vi "Yellow_Alarm_Counter.vi"(9 "Counter In":i32, 10 "Yellow Alarm":bool) -> (1 "Counter Out":i32, 2 "Counter Complete":bool)   [LabVIEW 2014]
panel:
  out "T Stoic Yellow \nMin Alarm":bool
  out "T Stoic Yellow \nMax Alarm":bool
  out "T Max Yellow\n Min Alarm":bool
  out "T Max Yellow \nMax Alarm":bool
  # "Yellow Alarm Counter Vi"
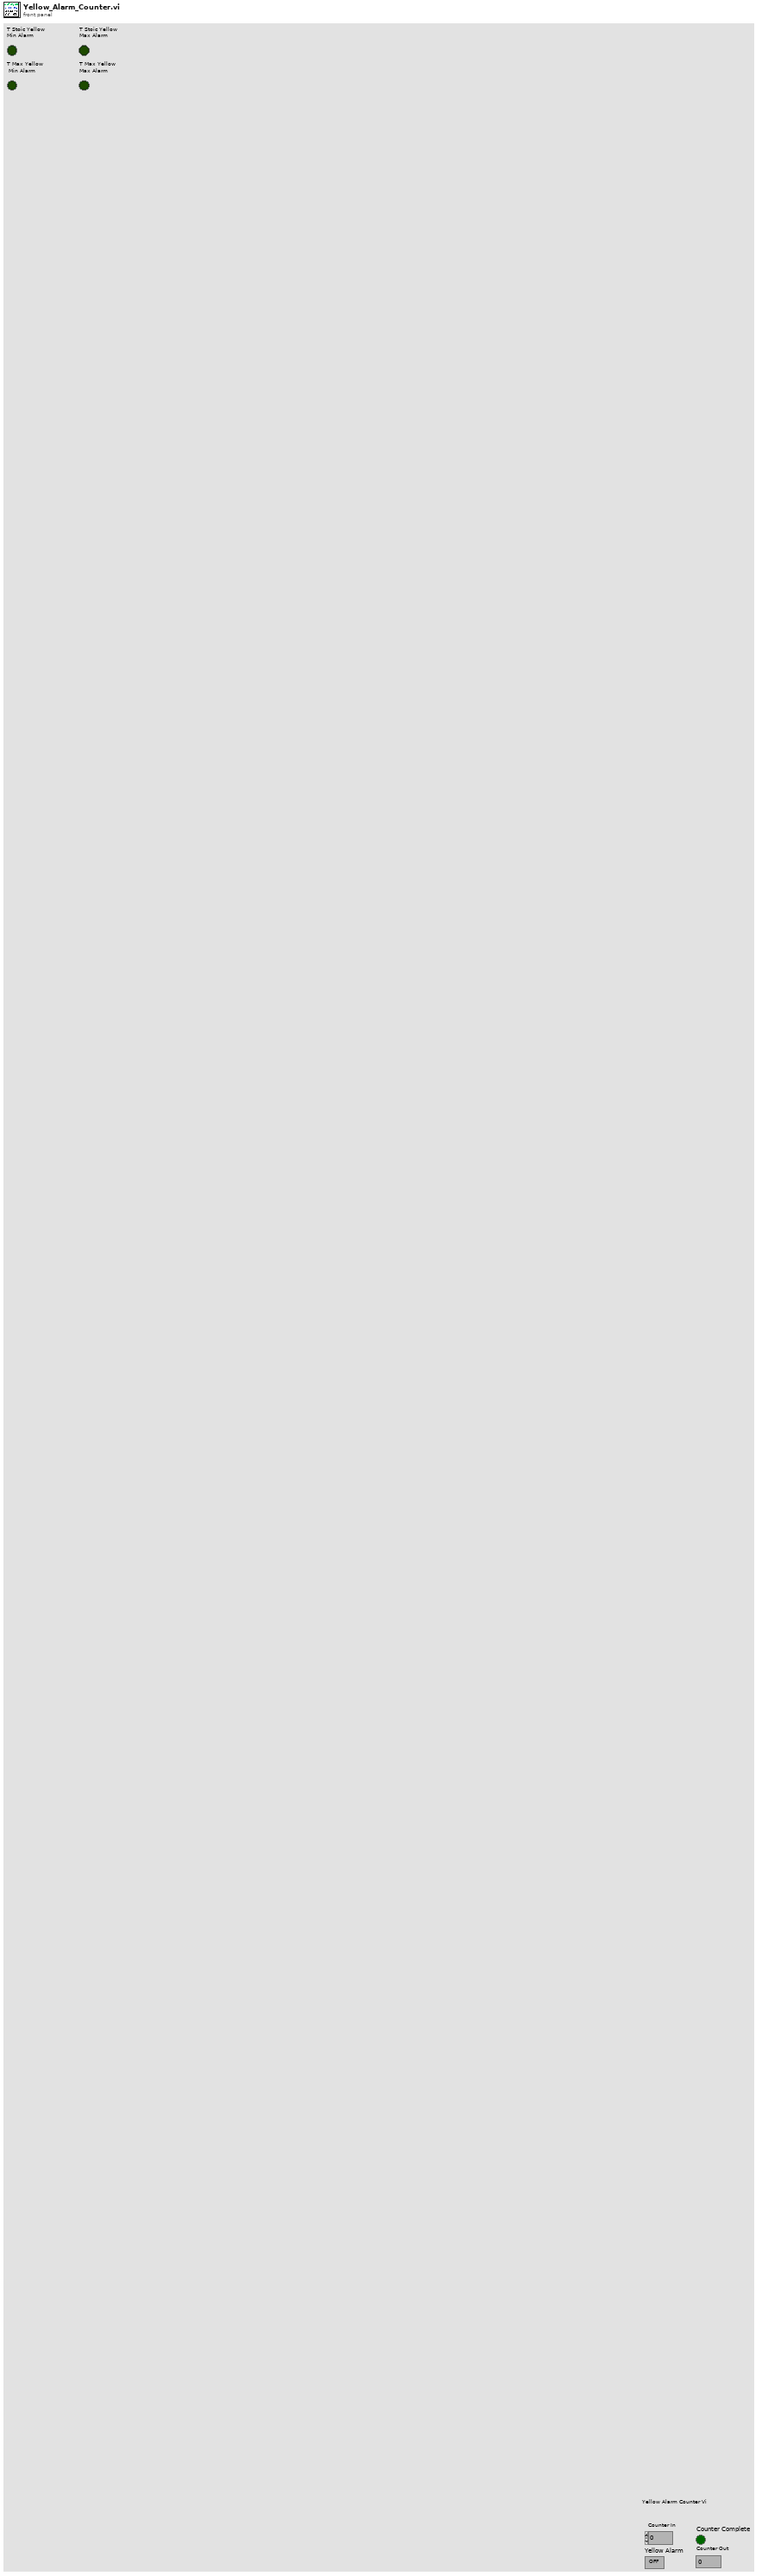
[diagram p1: front panel]
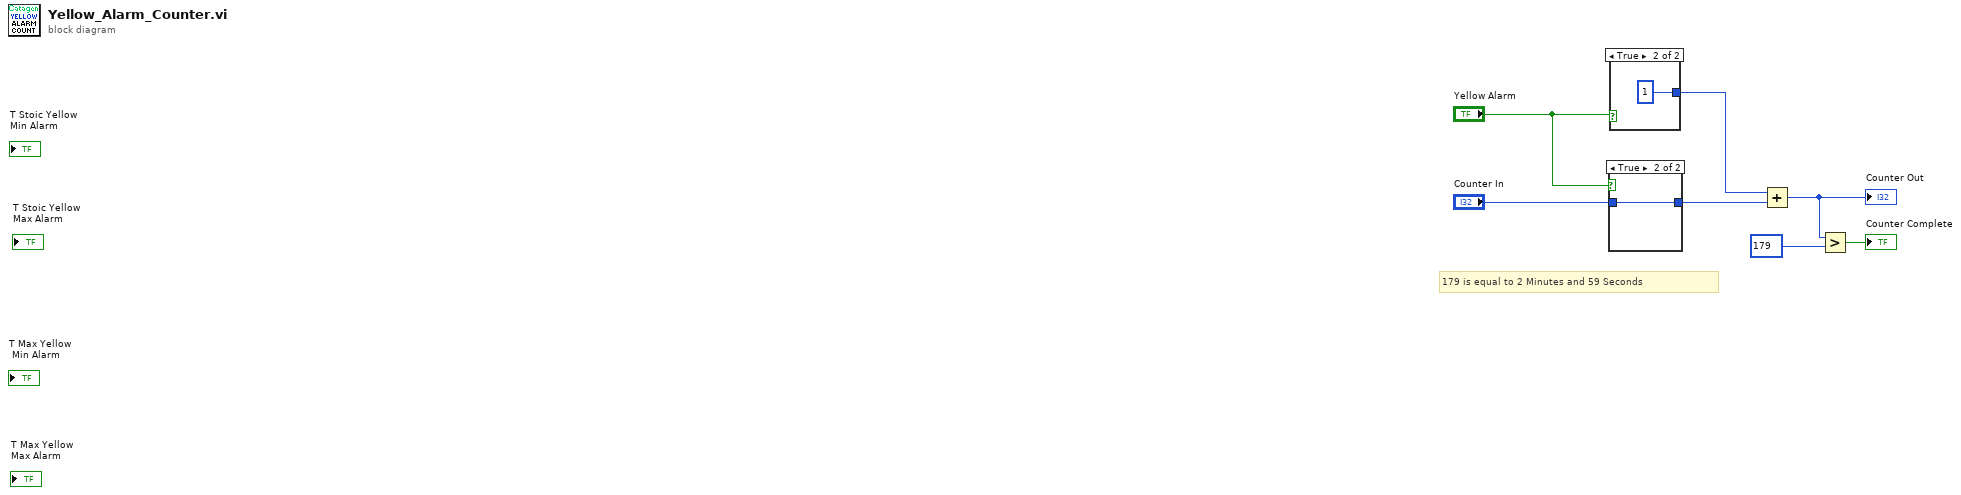
[diagram p0: block diagram]
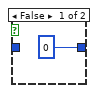
[diagram p2: hidden frame]
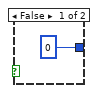
[diagram p3: hidden frame]
diagram:
  # "179 is equal to 2 Minutes and 59 Seconds"
  n1 = case shown="True" "Yellow Alarm" {
    tunnel: [0 w9] -> w5
    tunnel: "Counter In" -> [_ w9]
    frame False {
    }
    frame True {
    }
  }
  n2 = case shown="True" "Yellow Alarm" {
    tunnel: [0 1] -> w4
    frame False {
    }
    frame True {
    }
  }
  n3 = Add(x=w4, y=w5) -> (x+y=w7:i32)
  "Counter Out" <- w7
  n4 = Greater?(x=w7, y=179) -> (0:→"Counter Complete":bool)
